vi "cast_to_DoorInterface.vi"(0 "Object in":refnum<class "Timed Door.lvclass">, 5 "error in (no error)":errorcluster) -> (15 "Interface_object out":refnum<class "DoorInterface.lvclass">, 19 "error out":errorcluster)   [LabVIEW 2018, in "Timed Door.lvclass"]
doc: "Casts object to type of the interface and assign static method references. This method must be called only from corresponding methods belonging to the interface-applying classes."
uses:
  Timed Door.lvclass
  DoorInterface_interface/DoorInterface.lvclass
  DoorInterface_interface/method_refs.ctl
  util_DoorInterface_cls_Unlock.vi
  util_DoorInterface_cls_Lock.vi
  util_DoorInterface_cls_Is Door Open.vi
panel:
  # "Do not edit this method"
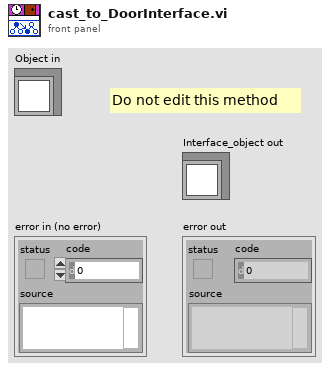
[diagram p1: front panel]
types:
  T1 = typedef "DoorInterface.lvclass/method_refs.ctl" = cluster{"Lock.vi":refnum<vi>, "Unlock.vi":refnum<vi>, "Is Door Open.vi":refnum<vi>}
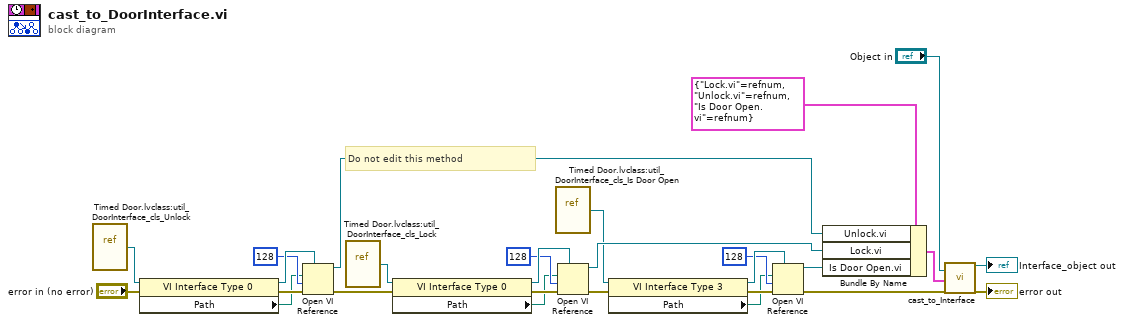
[diagram p0: block diagram]
diagram:
  # "Do not edit this method"
  n1 = vi-ref "Timed Door.lvclass:util_DoorInterface_cls_Unlock.vi"() -> (w22:refnum<vi>)
  n2 = property class="VI Interface Type 0"(reference=w22, error in="error in (no error)") -> (reference out=w19:refnum<vi>, error out=w18:errorcluster, "Path"=w16:path)
  n3 = Open VI Reference(type specifier VI Refnum (for type only)=w19, vi path=w16, options=128, error in (no error)=w18) -> (vi reference=w20:refnum<vi>, error out=w14:errorcluster)  [unwired: 2 in]
  n4 = vi-ref "Timed Door.lvclass:util_DoorInterface_cls_Lock.vi"() -> (w15:refnum<vi>)
  n5 = property class="VI Interface Type 0"(reference=w15, error in=w14) -> (reference out=w12:refnum<vi>, error out=w11:errorcluster, "Path"=w9:path)
  n6 = vi-ref "Timed Door.lvclass:util_DoorInterface_cls_Is Door Open.vi"() -> (w8:refnum<vi>)
  n7 = Open VI Reference(type specifier VI Refnum (for type only)=w12, vi path=w9, options=128, error in (no error)=w11) -> (vi reference=w13:refnum<vi>, error out=w7:errorcluster)  [unwired: 2 in]
  n8 = property class="VI Interface Type 3"(reference=w8, error in=w7) -> (reference out=w4:refnum<vi>, error out=w3:errorcluster, "Path"=w1:path)
  n9 = Open VI Reference(type specifier VI Refnum (for type only)=w4, vi path=w1, options=128, error in (no error)=w3) -> (vi reference=w5:refnum<vi>, error out=w6:errorcluster)  [unwired: 2 in]
  n10 = Bundle By Name(cluster=T1 {"Lock.vi"=refnum, "Unlock.vi"=refnum, "Is Door Open.vi"=refnum} ("method refs"), "Unlock.vi"=w20, "Lock.vi"=w13, "Is Door Open.vi"=w5) -> (w23:T1)
  n11 = call "cast_to_Interface.vi"("Object"="Object in", "method refs"=w23, "error in (no error)"=w6) -> ("Interface_object out"=→"Interface_object out":refnum<class "DoorInterface.lvclass">, "error out"=→"error out":errorcluster)  [unwired: 15 in]
